vi "GetStatus.vi"(1 "Elapsed Time":dbl, 2 "Num Hits":i32, 3 "Num Shots":i32) -> (0 "Status":string)   [LabVIEW 2015, in "Player.lvclass"]
uses:
  Player/Player.lvclass
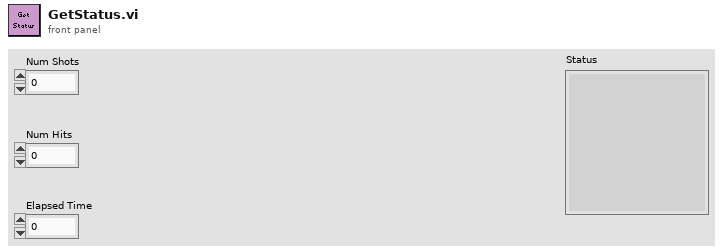
[diagram p1: front panel]
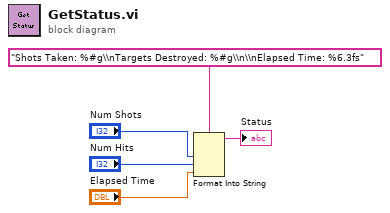
[diagram p0: block diagram]
diagram:
  n1 = Format Into String(format string="Shots Taken: %#g\\nTargets Destroyed: %#g\\n\\nElapsed Time: %6.3fs", "Num Shots", "Num Hits", "Elapsed Time") -> (resulting string=→"Status":string)  [unwired: 2 in, 1 out]
